vi "Sequence.Test.Print.Prepare.vi"(9 "Slot":T2, 10 "Code sets in":T3={"Ready"=FALSE, "DoubleOrder"=FALSE, "OrderDone"=FALSE, "AllowSingleSlot"=FALSE, "TunedA"=FALSE, "TunedB"=FALSE, "CheckDM"=FALSE, "ThresholdA"=0, "ThresholdB"=0, "Plate"=enum."Wabco", "ImgPath"=path "", "Variant"={"State"=enum."Init", "ImgPath"=path "", "WabcoPlate"="", "WabcoProduct"="", "ClientProduct"="", "ClientPlate"="", "TotalQuantity"=0, "OrderQuantity"=0, "Serial"=0, "Wabco"={"LaserJob"="", "AdditionalTxt"="037", "FactoryCode"="", "RevID"=0, "ForkID"=0, "FailuresLimit"=0, "GlobalCnt"=0, "Bank"=0, "SerialFormat"=enum."6 dig", "CoordA"={"X"=0.0, "Y"=0.0, "Angle"=0.0}, "CoordB"={"X"=0.0, "Y"=0.0, "Angle"=0.0}, "DMCconfig"=0}, "Client"={"LaserJob"="", "AdditionalTxt"="", "FactoryCode"="037", "RevID"=0, "ForkID"=0, "FailuresLimit"=0, "GlobalCnt"=0, "Bank"=0, "SerialFormat"=enum."6 dig", "CoordA"={"X"=0.0, "Y"=0.0, "Angle"=0.0}, "CoordB"={"X"=0.0, "Y"=0.0, "Angle"=0.0}, "DMCconfig"=0}}}) -> (0 "NextSerial":i32, 1 "Variables":string[](array[string]), 4 "JobSets":T1)   [LabVIEW 2016]
uses:
  Sequence.Code.Sets.ctl
  Sequence.PlateType.ctl
  Logger/Logger.Variant.Sets.ctl
  Station/Station.Changeover.State.vi
  Station/Station.Plate.Properties.ctl
  Sequence.Code.SerialFormat.ctl
  Drivers/V7310/LowLevel/V7310.Job.Sets.ctl
  Station/Station.ProductSlot.ctl
  Sequence.SerialsFglb.Action.ctl
  Drivers/V7310/LowLevel/V7310.Global.vi
  Station/Station.Global.vi
panel:
  out "TS":timestamp
  out "SN":string
  out "DataMatrix":string
  # "client - dol"
  # "client - gora"
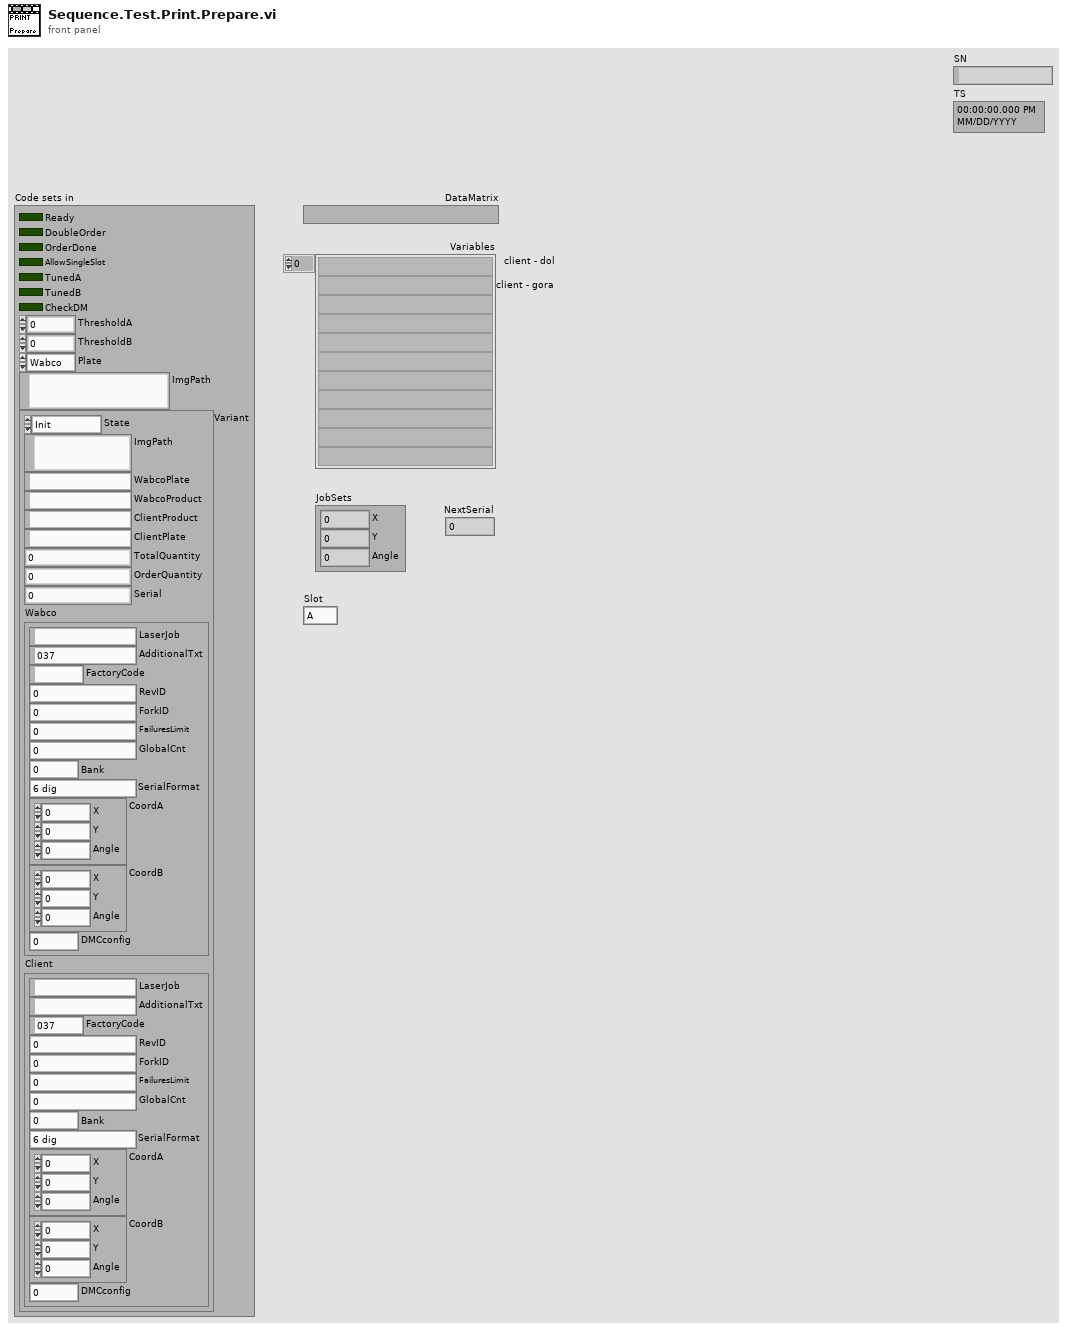
[diagram p1: front panel]
types:
  T1 = typedef "V7310.Job.Sets.ctl" = cluster{"X":dbl, "Y":dbl, "Angle":dbl}
  T2 = typedef "Station.ProductSlot.ctl" = enum8{"A", "B"}
  T3 = typedef "Sequence.Code.Sets.ctl" = cluster{"Ready":bool, "DoubleOrder":bool, "OrderDone":bool, "AllowSingleSlot":bool, "TunedA":bool, "TunedB":bool, "CheckDM":bool, "ThresholdA":u8, "ThresholdB":u8, "Plate":T4, "ImgPath":path, "Variant":T5}
  T4 = typedef "Sequence.PlateType.ctl" = enum16{"Wabco", "Client"}
  T5 = typedef "Logger.Variant.Sets.ctl" = cluster{"State":T6, "ImgPath":path, "WabcoPlate":string, "WabcoProduct":string, "ClientProduct":string, "ClientPlate":string, "TotalQuantity":u16, "OrderQuantity":u16, "Serial":i32, "Wabco":T7, "Client":T7}
  T6 = typedef "Station.Changeover.State.vi" = enum16{"Init", "Scaning", "NOK", "Wait for ack", "Ready"}
  T7 = typedef "Station.Plate.Properties.ctl" = cluster{"LaserJob":string, "AdditionalTxt":string, "FactoryCode":string, "RevID":u8, "ForkID":u8, "FailuresLimit":u16, "GlobalCnt":i32, "Bank":u8, "SerialFormat":T8, "CoordA":T1, "CoordB":T1, "DMCconfig":i32}
  T8 = typedef "Sequence.Code.SerialFormat.ctl" = enum8{"", "6 dig", "7 dig"}
  T9 = typedef "Sequence.SerialsFglb.Action.ctl" = enum16{"init", "get", "get next", "pass", "fail", "confirm", "clean"}
  T10 = typedef "V7310.Data.Status.ctl" = cluster{"State":T11, "LaserStatus":T12, "LaserStatusRaw":string, "Ref":refnum<k5>, "RTC TS":timestamp, "Conn TS":timestamp, "Msg":T13[], "JobInUse":string, "Jobs":string[], "Vars":T14[]}
  T11 = typedef "V7310.Data.Status.State.ctl" = enum16{"First", "Init", "Msg", "Error", "Abort", "Idle", "Run"}
  T12 = typedef "V7310.LaserStatus.ctl" = enum16{"-", "FatalError", "Initialize", "KeySwitchOpen", "TimeoutInterlock", "InterlockOpen", "StartUp", "ShutterlockOpen", "Standby", "Ready", "PrepareForMarking", "WaitForTrigger", "Marking"}
  T13 = typedef "V7310.Message.Data.ctl" = cluster{"ID":i32, "Msg":string}
  T14 = typedef "V7310.Job.Variable.ctl" = cluster{"Name":string, "Value":string}
  T15 = typedef "DMCConfiguatorGui.ConfigData.ctl" = cluster{"CreateDate":timestamp, "Name":string, "Components":T16[]}
  T16 = typedef "DMCConfiguatorGui.Component.ctl" = cluster{"Type":T17, "Var":T18, "Text":string}
  T17 = typedef "DMCConfiguatorGui.Type.ctl" = enum8{"Text", "Variable"}
  T18 = typedef "DMCConfiguatorGui.Var.ctl" = enum8{"-", "Wabco No", "Client No", "Serial", "Date"}
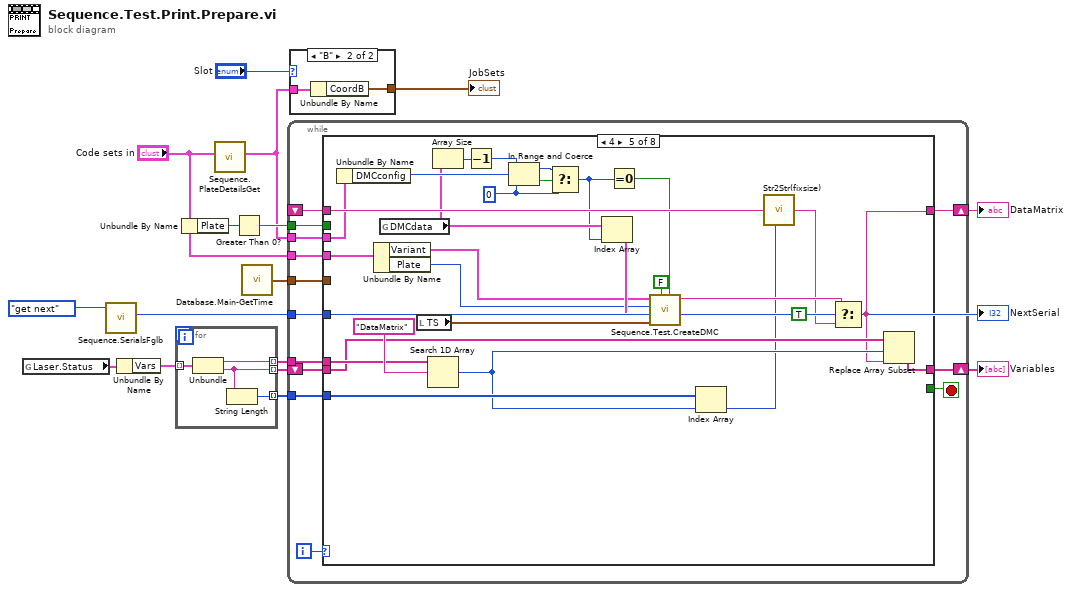
[diagram p0: block diagram]
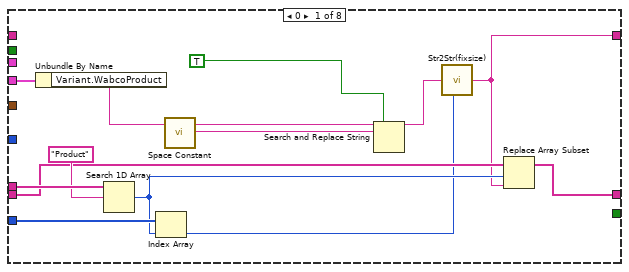
[diagram p2: hidden frame]
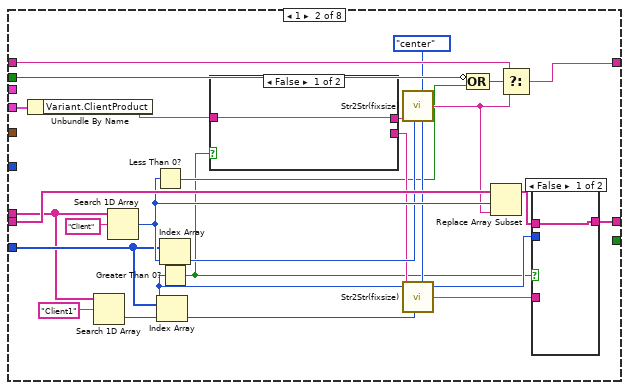
[diagram p3: hidden frame]
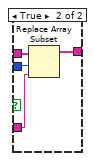
[diagram p4: hidden frame]
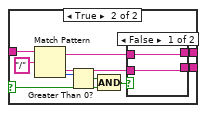
[diagram p5: hidden frame]
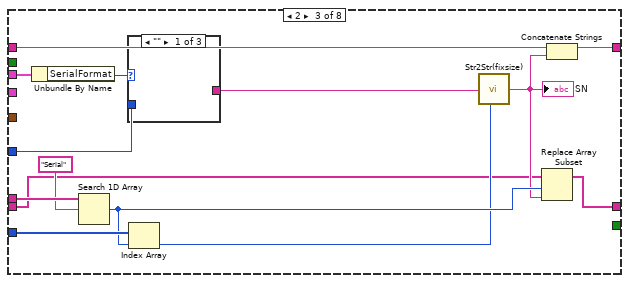
[diagram p7: hidden frame]
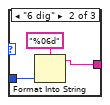
[diagram p8: hidden frame]
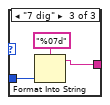
[diagram p9: hidden frame]
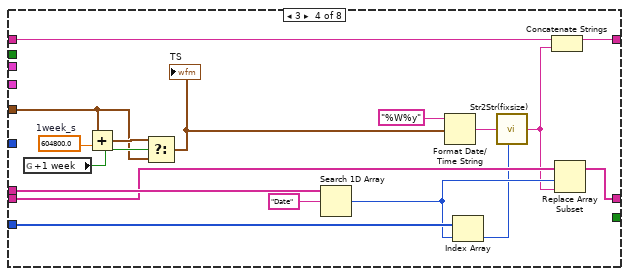
[diagram p10: hidden frame]
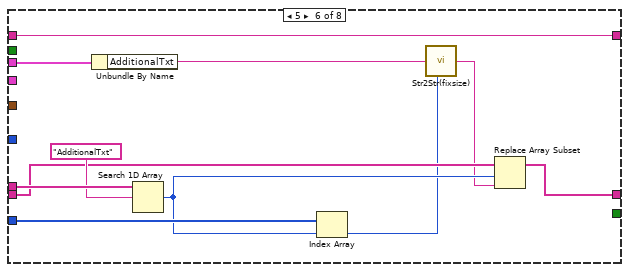
[diagram p11: hidden frame]
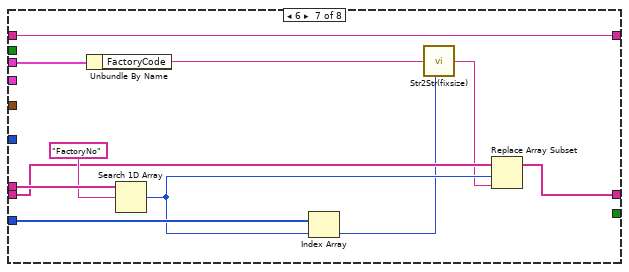
[diagram p12: hidden frame]
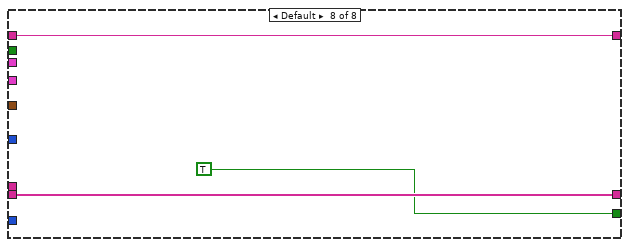
[diagram p13: hidden frame]
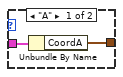
[diagram p14: hidden frame]
diagram:
  n1 = global read "V7310.Global.vi" "Laser.Status"() -> (w16:T10)
  n2 = call "Sequence.SerialsFglb.vi"("Action (get)"=Sequence.SerialsFglb.Action."get next" ("Action")) -> ("Serial out"=w12:i32)  [unwired: 6 in, 4 out]
  "NextSerial" <- w12
  n3 = Unbundle By Name(w16) -> ("Vars"=w15:T14[])
  n4 = for {
    tunnel: w15 -> [w20] mode=indexing
    tunnel: [w19] -> w14 mode=indexing
    tunnel: [w18] -> w13 mode=indexing
    tunnel: [w17] -> w7 mode=indexing
    n5 = Unbundle(w20) -> ("Name"=w19:string, "Value"=w18:string)
    n6 = String Length(string=w18) -> (length=w17:i32)
  }
  n7 = Unbundle By Name("Code sets in") -> ("Plate"=w6:T4)
  n8 = call "Sequence.PlateDetailsGet.vi"("Code in"="Code sets in") -> ("PlateDetails"=w4:T7)  [unwired: 9 in, 1 out]
  n9 = Greater Than 0?(x=w6) -> (x > 0?=w5:bool)
  n10 = call "Database.Main-GetTime.vi"() -> ("TS"=w1:timestamp)  [unwired: 1 in]
  n11 = while {
    tunnel: w4 -> [w33]
    tunnel: w14 -> [w32]
    shift-right: [w30] -> w11
    shift-left: w13 -> [w31]
    tunnel: w12 -> [w28]
    shift-right: [w26] -> w10
    shift-left: _ -> [w25]
    tunnel: "Code sets in" -> [w24]
    tunnel: w5 -> [w23]
    tunnel: w7 -> [w22]
    tunnel: w1 -> [w21]
    i -> [w29]
    stop <- w27 stop-if-true
    n12 = case shown="4" w29 {
      tunnel: w33 -> [_ _ w101 _ w139 w167 w178 _]
      tunnel: w32 -> [w46 w59 w104 w127 w155 w166 w177 _]
      tunnel: w31 -> [w39 w64 w91 w121 w152 w162 w175 w181]
      tunnel: [w34 w52 w92 w125 w132 w164 w174 w181] -> w30
      tunnel: w28 -> [_ _ w102 _ w141 _ _ _]
      tunnel: [_ _ _ _ _ _ _ TRUE] -> w27
      tunnel: [w35 w65 w98 w123 w148 w163 w173 w179] -> w26
      tunnel: w25 -> [_ w66 w99 w122 w154 w163 w173 w179]
      tunnel: w24 -> [w42 w69 _ _ w145 _ _ _]
      tunnel: w23 -> [_ w68 _ _ _ _ _ _]
      tunnel: w22 -> [w38 w60 w97 w120 w153 w160 w172 _]
      tunnel: w21 -> [_ _ _ w111 _ _ _ _]
      frame 0 {
        n13 = Unbundle By Name(w42) -> ("Variant.WabcoProduct"=w41:string)
        n14 = Search 1D Array(1D array=w46, element="Product") -> (index of element=w37:i32)  [unwired: 1 in]
        n15 = Index Array(array=w38, index=w37) -> (element=w36:i32)
        n16 = call <vilib>:"Space Constant.vi"() -> ("String"=w44:string)
        n17 = Search and Replace String(replace all?=TRUE ("replace all? (F)"), input string=w41, search string=w44) -> (result string=w40:string)  [unwired: 5 in, 3 out]
        n18 = call "Str2Str(fixsize).vi"("string"=w40, "size"=w36) -> ("fixed size string"=w35:string)  [unwired: 1 in]
        n19 = Replace Array Subset(array=w39, new element=w35, index=w37) -> (w34:string[])
      }
      frame 1 {
        w57 = enum16{"left", "right", "center"}."center" ("justify (left)")
        n20 = Unbundle By Name(w69) -> ("Variant.ClientProduct"=w49:string)
        n21 = Search 1D Array(1D array=w59, element="Client1") -> (index of element=w51:i32)  [unwired: 1 in]
        n22 = Search 1D Array(1D array=w59, element="Client") -> (index of element=w63:i32)  [unwired: 1 in]
        n23 = Less Than 0?(x=w63) -> (x < 0?=w48:bool)
        n24 = Index Array(array=w60, index=w51) -> (element=w54:i32)
        n25 = Index Array(array=w60, index=w63) -> (element=w62:i32)
        n26 = Greater Than 0?(x=w51) -> (x > 0?=w47:bool)
        n27 = case shown="False" w47 {
          selector: w47 -> [_ w77]
          tunnel: w49 -> [w76 w86]
          tunnel: [w76 w84] -> w56
          tunnel: [_ w82] -> w55
          frame False {
          }
          frame True {
            n28 = Match Pattern(string=w86, regular expression="/") -> (before substring=w81:string, after substring=w83:string, offset past match=w80:i32)  [unwired: 1 in, 1 out]
            n29 = Greater Than 0?(x=w80) -> (x > 0?=w79:bool)
            n30 = Compound Arithmetic op=AND(w79, w77) -> (w78:bool)
            n31 = case shown="False" w78 {
              tunnel: [w88 w90] -> w84
              tunnel: w83 -> [w87 w90]
              tunnel: [w87 w89] -> w82
              tunnel: w81 -> [w88 w89]
              frame False {
              }
              frame True {
              }
            }
          }
        }
        n32 = call "Str2Str(fixsize).vi"("string"=w56, "size"=w62, "justify (left)"=w57) -> ("fixed size string"=w61:string)
        n33 = call "Str2Str(fixsize).vi"("string"=w55, "size"=w54, "justify (left)"=w57) -> ("fixed size string"=w53:string)
        n34 = Compound Arithmetic op=OR(invert w68, w48) -> (w67:bool)
        n35 = Replace Array Subset(array=w64, new element=w61, index=w63) -> (w50:string[])
        n36 = Select(t=w66, s=w67, f=w61) -> (s? t:f=w65:string)
        n37 = case shown="False" w47 {
          tunnel: w50 -> [w71 w75]
          tunnel: w53 -> [_ w74]
          tunnel: [w71 w73] -> w52
          tunnel: w51 -> [_ w72]
          frame False {
          }
          frame True {
            n38 = Replace Array Subset(array=w75, new element=w74, index=w72) -> (w73:string[])
          }
        }
      }
      frame 2 {
        n39 = Unbundle By Name(w101) -> ("SerialFormat"=w100:T8)
        n40 = Search 1D Array(1D array=w104, element="Serial") -> (index of element=w96:i32)  [unwired: 1 in]
        n41 = case shown="\"\"" w100 {
          tunnel: w102 -> [_ w107 w110]
          tunnel: [_ w105 w108] -> w95
          frame "" {
          }
          frame "6 dig" {
            n42 = Format Into String(format string="%06d", w107) -> (resulting string=w105:string)  [unwired: 2 in, 1 out]
          }
          frame "7 dig" {
            n43 = Format Into String(format string="%07d", w110) -> (resulting string=w108:string)  [unwired: 2 in, 1 out]
          }
        }
        n44 = Index Array(array=w97, index=w96) -> (element=w94:i32)
        n45 = call "Str2Str(fixsize).vi"("string"=w95, "size"=w94) -> ("fixed size string"=w93:string)  [unwired: 1 in]
        "SN" <- w93
        n46 = Replace Array Subset(array=w91, new element=w93, index=w96) -> (w92:string[])
        n47 = Concatenate Strings(w99, w93) -> (w98:string)
      }
      frame 3 {
        w115 = 604800.0  # 1week_s
        n48 = global read "Station.Global.vi" "+1 week"() -> (w113:bool)
        n49 = Add(x=w111, y=w115) -> (x+y=w114:timestamp)
        n50 = Select(t=w114, s=w113, f=w111) -> (s? t:f=w112:timestamp)
        "TS" <- w112
        n51 = Search 1D Array(1D array=w127, element="Date") -> (index of element=w119:i32)  [unwired: 1 in]
        n52 = Format Date/Time String(time format string (%c)="%W%y", seconds (now)=w112) -> (date/time string=w118:string)  [unwired: 1 in]
        n53 = Index Array(array=w120, index=w119) -> (element=w117:i32)
        n54 = call "Str2Str(fixsize).vi"("string"=w118, "size"=w117) -> ("fixed size string"=w116:string)  [unwired: 1 in]
        n55 = Concatenate Strings(w122, w116) -> (w123:string)
        n56 = Replace Array Subset(array=w121, new element=w116, index=w119) -> (w125:string[])
      }
      frame 4 {
        w133 = 0 ("x")
        n57 = Unbundle By Name(w139) -> ("DMCconfig"=w137:i32)
        n58 = Unbundle By Name(w145) -> ("Variant"=w142:T5, "Plate"=w143:T4)
        n59 = global read "Station.Global.vi" "DMCdata"() -> (w129:T15[])
        n60 = local read "TS"() -> (w146:timestamp)
        n61 = Search 1D Array(1D array=w155, element="DataMatrix") -> (index of element=w151:i32)  [unwired: 1 in]
        n62 = Array Size(array=w129) -> (size(s)=w138:i32)
        n63 = Decrement(x=w138) -> (x-1=w136:i32)
        n64 = In Range and Coerce(upper limit=w136, x=w137, lower limit=w133) -> (coerced(x)=w134:i32, In Range?=w135:bool)
        n65 = Select(t=w134, s=w135, f=w133) -> (s? t:f=w128:i32)
        n66 = Index Array(array=w129, index=w128) -> (element=w144:T15)
        n67 = Equal To 0?(x=w128) -> (x = 0?=w131:bool)
        n68 = call "Sequence.Test.CreateDMC.vi"("Default"=w131, "TS (now)"=w146, "GUI? (F)"=FALSE, "Serial (0)"=w141, "DMCConfig"=w144, "Plate"=w143, "Variant"=w142) -> ("DMC"=w150:string)  [unwired: 3 in, 1 out]
        n69 = Index Array(array=w153, index=w151) -> (element=w147:i32)
        n70 = call "Str2Str(fixsize).vi"("string"=w154, "size"=w147) -> ("fixed size string"=w149:string)  [unwired: 1 in]
        n71 = Select(t=w150, s=TRUE, f=w149) -> (s? t:f=w148:string)
        n72 = Replace Array Subset(array=w152, new element=w148, index=w151) -> (w132:string[])
      }
      frame 5 {
        n73 = Unbundle By Name(w167) -> ("AdditionalTxt"=w161:string)
        n74 = Search 1D Array(1D array=w166, element="AdditionalTxt") -> (index of element=w159:i32)  [unwired: 1 in]
        n75 = Index Array(array=w160, index=w159) -> (element=w158:i32)
        n76 = call "Str2Str(fixsize).vi"("string"=w161, "size"=w158) -> ("fixed size string"=w157:string)  [unwired: 1 in]
        n77 = Replace Array Subset(array=w162, new element=w157, index=w159) -> (w164:string[])
      }
      frame 6 {
        n78 = Unbundle By Name(w178) -> ("FactoryCode"=w169:string)
        n79 = Search 1D Array(1D array=w177, element="FactoryNo") -> (index of element=w171:i32)  [unwired: 1 in]
        n80 = Index Array(array=w172, index=w171) -> (element=w170:i32)
        n81 = call "Str2Str(fixsize).vi"("string"=w169, "size"=w170) -> ("fixed size string"=w168:string)  [unwired: 1 in]
        n82 = Replace Array Subset(array=w175, new element=w168, index=w171) -> (w174:string[])
      }
      frame Default {
      }
    }
  }
  "Variables" <- w11
  "DataMatrix" <- w10
  n83 = case shown="\"B\"" "Slot" {
    tunnel: w4 -> [w183 w185]
    tunnel: [w182 w184] -> w8
    frame "A" {
      n84 = Unbundle By Name(w183) -> ("CoordA"=w182:T1)
    }
    frame "B" {
      n85 = Unbundle By Name(w185) -> ("CoordB"=w184:T1)
    }
  }
  "JobSets" <- w8
